vi "RtdeAddOutput.vi"(8 "Index for registers":i32, 9 "Data":i32(ring) items=["Timestamp", "TargetQ", "TargetQd", "TargetQdd", "TargetCurrent", "TargetMoment", "ActualQ", "ActualQd", "ActualCurrent", "JointControlOutput", "ActualTcpPose", "ActualTcpSpeed", "ActualTcpForce", "TargetTcpPose", "TargetTcpSpeed", "ActualDigitalInputBits", "JointTemperatures", "ActualExecutionTime", "RobotMode", "JointMode", "SafetyMode", "SafetyStatus", "ActualToolAccelerometer", "SpeedScaling", "TargetSpeedFraction", "ActualMomentum", "ActualMainVoltage", "ActualRobotVoltage", "ActualRobotCurrent", "ActualJointVoltage", "ActualDigitalOutputBits", "RuntimeState", "ElbowPosition", "ElbowVelocity", "RobotStatusBits", "SafetyStatusBits", "AnalogIOTypes", "StandardAnalogInput0", "StandardAnalogInput1", "StandardAnalogOutput0", "StandardAnalogOutput1", "IOCurrent", "Euromap67InputBits", "Euromap67OutputBits", "Euromap67_24VVoltage", "Euromap67_24VCurrent", "ToolMode", "ToolAnalogInputTypes", "ToolAnalogInput0", "ToolAnalogInput1", "ToolOutputVoltage", "ToolOutputCurrent", "ToolTemperature", "TcpForceScalar", "OutputBitRegisters0To31", "OutputBitRegisters32To63", "OutputBitRegisters", "OutputIntRegisters", "OutputDoubleRegisters", "InputBitRegisters0To31", "InputBitRegisters32To63", "InputBitRegisters", "InputIntRegisters", "InputDoubleRegisters", "ToolOutputMode", "ToolDigitalOutput0mode", "ToolDigitalOutput1Mode", "Payload", "PayloadCOG", "PayloadInertia", "ScriptControlLine", "FTRawWrench"], 10 "RTDE Connect Parameters":refnum<k24>, 11 "error in":errorcluster) -> (2 "RTDE Connect Parameters":refnum<k24>, 3 "error out":errorcluster)   [LabVIEW 2016, in "UnderAutomation.UniversalRobots.lvlib"]
uses:
  UnderAutomation.UniversalRobots.lvlib
  C:/Users/fg/Documents/UniversalRobots.vi/LabVIEW_2024/UnderAutomation.UniversalRobots/lib/UnderAutomation.UniversalRobots.dll
  LabVIEW_2024/UnderAutomation.UniversalRobots/lib/UnderAutomation.UniversalRobots.dll
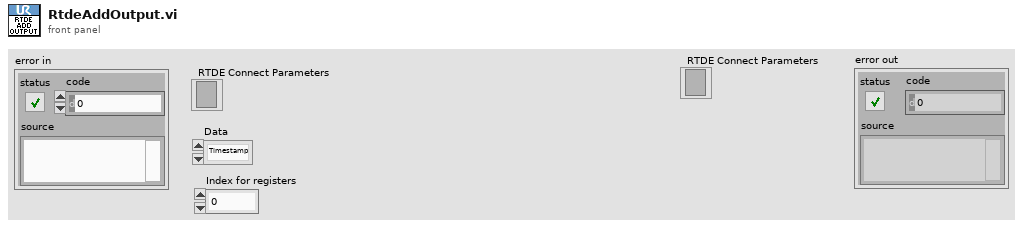
[diagram p1: front panel]
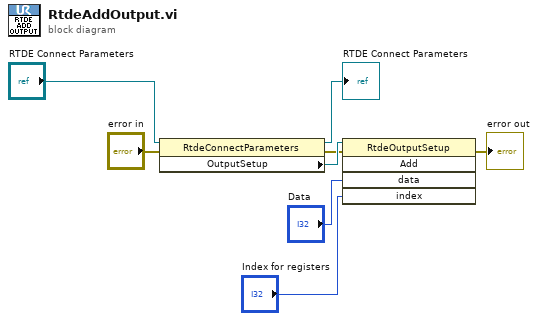
[diagram p0: block diagram]
diagram:
  n1 = property class="RtdeConnectParameters"(reference="RTDE Connect Parameters", error in="error in") -> (reference out=→"RTDE Connect Parameters":refnum<k24>, error out=w1:errorcluster, "OutputSetup"=w5:refnum<k24>)
  n2 = invoke class="RtdeOutputSetup" method="Add"(reference=w5, error in=w1, "data"="Data", "index"="Index for registers") -> (error out=→"error out":errorcluster)  [unwired: 1 in, 4 out]
